vi "test.runner.top.vi"() -> ()   [LabVIEW 2020]
panel:
  out "Name":string
  out "size(s)":i32
  out "data":bool
  out "Array":path[](array[path])
  out "error out":errorcluster
  in  "error in":errorcluster
  out "directory":bool
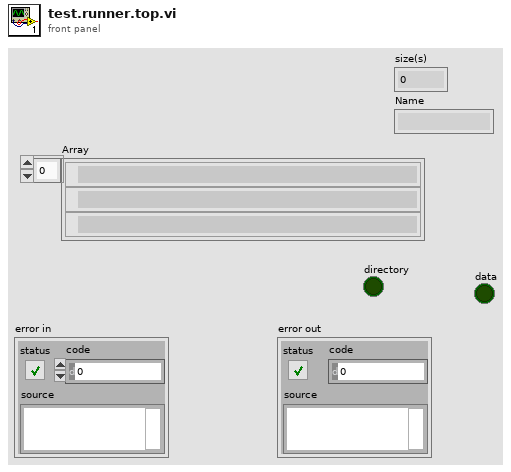
[diagram p1: front panel]
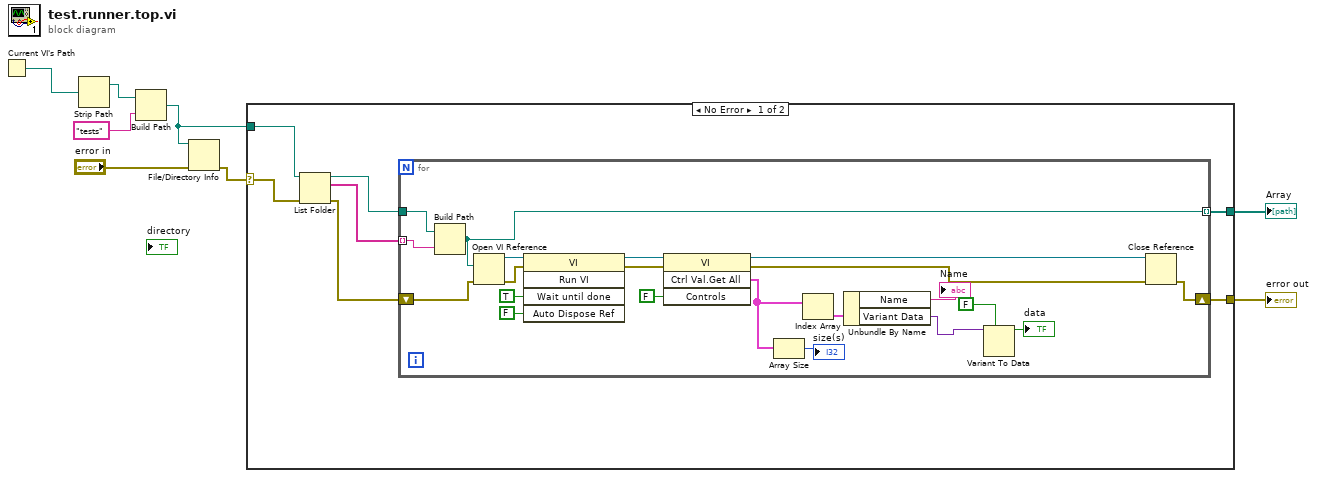
[diagram p0: block diagram]
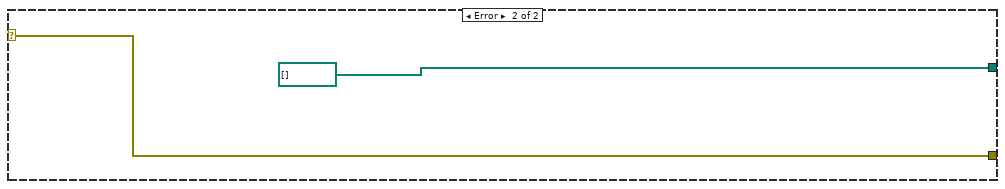
[diagram p2: hidden frame]
diagram:
  n1 = Current VI's Path() -> (path=w6:path)
  n2 = Strip Path(path=w6) -> (stripped path=w5:path)  [unwired: 1 out]
  n3 = Build Path(base path=w5, name or relative path="tests") -> (appended path=w3:path)
  n4 = File/Directory Info(path=w3, error in="error in") -> (error out=w4:errorcluster)  [unwired: 6 out]
  n5 = case shown="No Error" w4 {
    selector: w4 -> [w14 w37]
    tunnel: w3 -> [w15 _]
    tunnel: [w12 path[] []] -> w2
    tunnel: [w10 w37] -> w1
    frame No Error {
      n6 = List Folder(path=w15, error in=w14) -> (path out=w13:path, filenames=w9:string[], error out=w11:errorcluster)  [unwired: 2 in, 1 out]
      n7 = for {
        tunnel: [w34] -> w12 mode=indexing
        tunnel: w13 -> [w36]
        shift-right: [w31] -> w10
        shift-left: w11 -> [w33]
        tunnel: w9 -> [w35] mode=indexing
        n8 = Build Path(base path=w36, name or relative path=w35) -> (appended path=w34:path)
        n9 = Open VI Reference(vi path=w34, error in (no error)=w33) -> (vi reference=w32:refnum<vi>, error out=w30:errorcluster)  [unwired: 4 in]
        n10 = invoke class="VI" method="Run VI"(reference=w32, error in=w30, "Wait until done"=TRUE ("Wait Until Done"), "Auto Dispose Ref"=FALSE ("Auto Dispose Reference")) -> (reference out=w29:refnum<vi>, error out=w24:errorcluster)  [unwired: 1 in, 3 out]
        n11 = invoke class="VI" method="Ctrl Val.Get All"(reference=w29, error in=w24, "Controls"=FALSE) -> (reference out=w25:refnum<vi>, error out=w23:errorcluster, "Get All Control Values Variant"=w18:cluster{"Name":string, "Variant Data":variant}[])  [unwired: 1 in, 1 out]
        n12 = Array Size(array=w18) -> (size(s)=→"size(s)":i32)
        n13 = Index Array(array=w18) -> (element=w22:cluster{"Name":string, "Variant Data":variant})  [unwired: 1 in]
        n14 = Unbundle By Name(w22) -> ("Name"=→"Name":string, "Variant Data"=w21:variant)
        n15 = Variant To Data(type=FALSE, Variant=w21) -> (data=→"data":bool)  [unwired: 1 in, 1 out]
        n16 = Close Reference(reference=w25, error in (no error)=w23) -> (error out=w31:errorcluster)
      }
    }
    frame Error {
    }
  }
  "error out" <- w1
  "Array" <- w2
